vi "Configure Function.vi"(7 "Function":u16(ring) items=["DCI", "DCV"], 8 "error in (no error)":errorcluster, 11 "HP 3457A in":refnum<class "HP 3457A.lvclass">) -> (0 "error out":errorcluster, 3 "HP 3457A out":refnum<class "HP 3457A.lvclass">)   [LabVIEW 2020, in "HP 3457A.lvclass"]
uses:
  HP 3457A.lvclass
  C:/Sandbox/RF Bench/Source Code/WiSpry Test Framework/Instruments/Instrument.lvclass
  C:/Sandbox/RF Bench/Source Code/WiSpry Test Framework/Instruments/Digital Multimeter/Digital Multimeter.lvclass
  Instrument.lvclass/Instrument.ctl
  Digital Multimeter.lvclass/Digital Multimeter.ctl
  Instrument.lvclass
  Digital Multimeter.lvclass
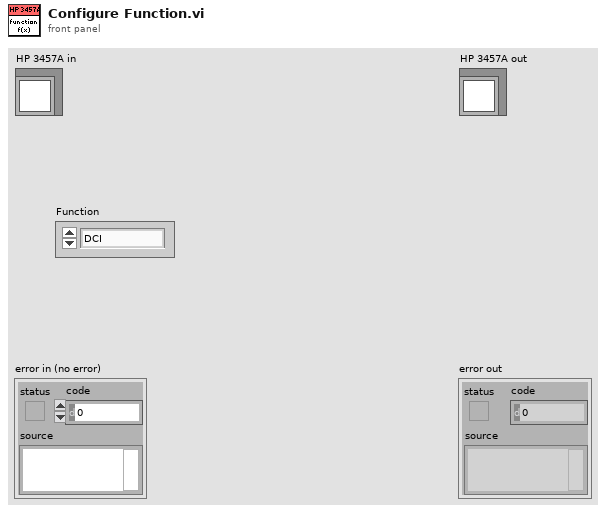
[diagram p1: front panel]
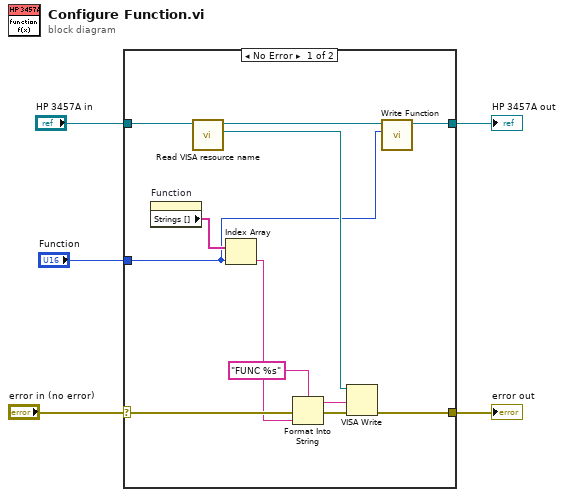
[diagram p0: block diagram]
diagram:
  n1 = case shown="No Error" "error in (no error)" {
    selector: "error in (no error)" -> [w15 w19]
    tunnel: "HP 3457A in" -> [w17 w18]
    tunnel: [w9 w19] -> w3
    tunnel: [w6 w18] -> w2
    tunnel: "Function" -> [w8 _]
    frame No Error {
      n2 = property on="Function" class="Ring (strict)"() -> ("Strings []"=w14:string[])  [unwired: 2 in, 2 out]
      n3 = call "Read VISA resource name.vi"("Instrument in"=w17) -> ("VISA resource name"=w10:refnum<visa-resource-name>, "Instrument out"=w7:refnum<class "HP 3457A.lvclass">)  [unwired: 9 in]
      n4 = Index Array(array=w14, index=w8) -> (element=w13:string)
      n5 = Format Into String(format string="FUNC %s", error in=w15, w13) -> (resulting string=w11:string, error out=w12:errorcluster)  [unwired: 1 in]
      n6 = VISA Write(VISA resource name=w10, write buffer=w11, error in (no error)=w12) -> (error out=w9:errorcluster)  [unwired: 2 out]
      n7 = call "Write Function.vi"("Function"=w8, "Digtal Multimeter in"=w7) -> ("Digtal Multimeter out"=w6:refnum<class "HP 3457A.lvclass">)  [unwired: 9 in]
    }
    frame Error {
    }
  }
  "error out" <- w3
  "HP 3457A out" <- w2
